vi "Get CHM Path.vi"() -> (0 "appended path":path)   [LabVIEW 2020, in "Modbus Master System Explorer.lvlib"]
uses:
  Modbus Master System Explorer.lvlib
  Shared/Constants.vi
  Shared/Modbus Master Shared.lvlib
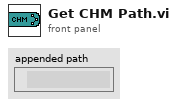
[diagram p1: front panel]
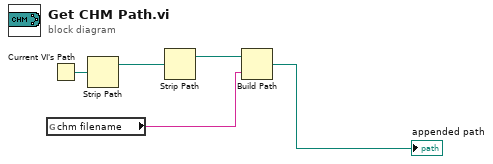
[diagram p0: block diagram]
diagram:
  n1 = global read "Constants.vi" "chm filename"() -> (w5:string)
  n2 = Current VI's Path() -> (path=w3:path)
  n3 = Strip Path(path=w3) -> (stripped path=w2:path)  [unwired: 1 out]
  n4 = Strip Path(path=w2) -> (stripped path=w1:path)  [unwired: 1 out]
  n5 = Build Path(base path=w1, name or relative path=w5) -> (appended path=→"appended path":path)
